vi "EF_DAQThread.vi"(9 "EF_DAQThread_Data":T1, 10 "EF_AllQRefs":T3, 11 "Exit":refnum<user-event>) -> ()   [LabVIEW 2017]
uses:
  Types/EF_AllQRefs.ctl
  Types/EF_GUIThread_QRef.ctl
  Types/EF_GUIThread_QData.ctl
  Types/EF_GUIThread_QCmds.ctl
  Types/EF_DAQThread_QRef.ctl
  Types/EF_DAQThread_QData.ctl
  Types/EF_DAQThread_QCmds.ctl
  Types/EF_DataProcThread_QRef.ctl
  Types/EF_DataProcThread_QData.ctl
  Types/EF_DataProcThread_QCmds.ctl
  Types/EF_AnalysisThread_QRef.ctl
  Types/EF_AnalysisThread_QData.ctl
  Types/EF_AnalysisThread_QCmds.ctl
  Types/EF_DAQThread_Data.ctl
  _lib/PQ/PicoHarp/PH_InitInfo.ctl
  _lib/PQ/PicoHarp/PH_MeasMode.ctl
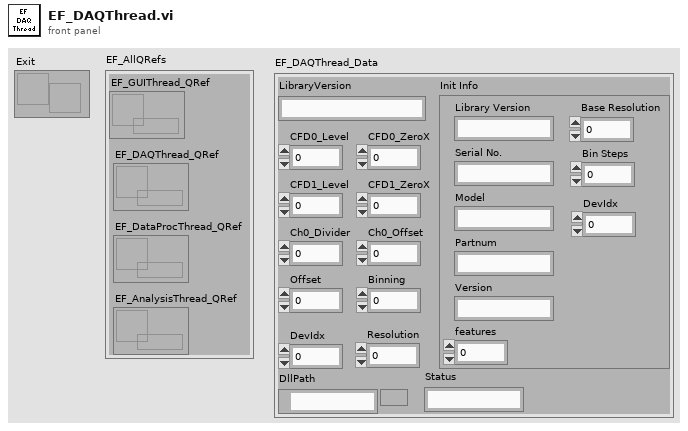
[diagram p1: front panel]
types:
  T1 = typedef "EF_DAQThread_Data.ctl" = cluster{"LibraryVersion":string, "CFD0_Level":i32, "CFD0_ZeroX":i32, "CFD1_Level":i32, "CFD1_ZeroX":i32, "Ch0_Divider":i32, "Ch0_Offset":i32, "Init Info":T2, "DevIdx":i32, "Offset":i32, "Binning":i32, "Resolution":dbl, "DllPath":path, "Status":string}
  T2 = typedef "PH_InitInfo.ctl" = cluster{"Library Version":string, "Serial No.":string, "Model":string, "Partnum":string, "Version":string, "features":i32, "Base Resolution":dbl, "Bin Steps":i32, "DevIdx":i32}
  T3 = typedef "EF_AllQRefs.ctl" = cluster{"EF_GUIThread_QRef":T4, "EF_DAQThread_QRef":T5, "EF_DataProcThread_QRef":T6, "EF_AnalysisThread_QRef":T7}
  T4 = typedef "EF_GUIThread_QRef.ctl" = refnum<queue>
  T5 = typedef "EF_DAQThread_QRef.ctl" = refnum<queue>
  T6 = typedef "EF_DataProcThread_QRef.ctl" = refnum<queue>
  T7 = typedef "EF_AnalysisThread_QRef.ctl" = refnum<queue>
  T8 = typedef "EF_DAQThread_QData.ctl" = cluster{"EF_DAQThread_Cmds":T9, "Parameter":i32[], "error in (no error)":errorcluster}
  T9 = typedef "EF_DAQThread_QCmds.ctl" = enum16{"Idle", "Init", "InitHW", "SetCFD0", "SetCFD1", "SetCh0Divider", "SetCh0Offset", "SetOffset", "SetBinning", "GetResolution", "GetRates", "StartMeas", "ReadFiFo", "StopMeas", "WriteStatus", "_Error_", "Exit"}
  T10 = typedef "EF_AnalysisThread_QData.ctl" = cluster{"Cmd":T11, "Histo":u32[], "DecayT0":dbl, "HistoRes":dbl, "TotalBinHistStart":u64, "TimeTraceRes":dbl, "Total bin":u64, "TickCount":u32, "LTThreshold":dbl, "TTLActivate":bool, "TTLDelay":dbl, "TTLWidth":dbl, "MinIntCounts":u32}
  T11 = typedef "EF_AnalysisThread_QCmds.ctl" = enum16{"Exit", "CalcAvgLT", "CalcDelay", "SetDecayT0", "SetHistoRes", "SetTimeTraceRes", "SetLTThreshold", "SetTTLActiv", "SetTTLDelay", "SetTTLWidth", "SetMinIntCounts"}
  T12 = typedef "EF_GUIThread_QData.ctl" = cluster{"Histo":u32[], "Rates":i32[], "Cmd":T13, "Res":dbl, "TimeTrace":u32[], "Bin":i32, "Status":string, "Total bin":u64, "AvgLTs":dbl[], "TotalBinsHistStart":u64[], "HistStartTimes":dbl[], "MinDelays":dbl[], "ShortDelay":bool, "Pending TTLs":i32, "error in (no error)":errorcluster, "DeltaT":dbl, "NumLTs":i32}
  T13 = typedef "EF_GUIThread_QCmds.ctl" = enum16{"_none_", "Res", "Histo", "TTrace", "Lifetime", "Rates", "Status", "ShortDelay", "_Error_"}
  T14 = typedef "EF_DataProcThread_QData.ctl" = cluster{"EF_DataProc_Cmds":T15, "nActual":i32, "Buffer":u32[], "TickCount":u32, "Param":i32}
  T15 = typedef "EF_DataProcThread_QCmds.ctl" = enum16{"Exit", "Proc", "Init", "SetShift", "SetThres"}
  T16 = typedef "PH_MeasMode.ctl" = i32
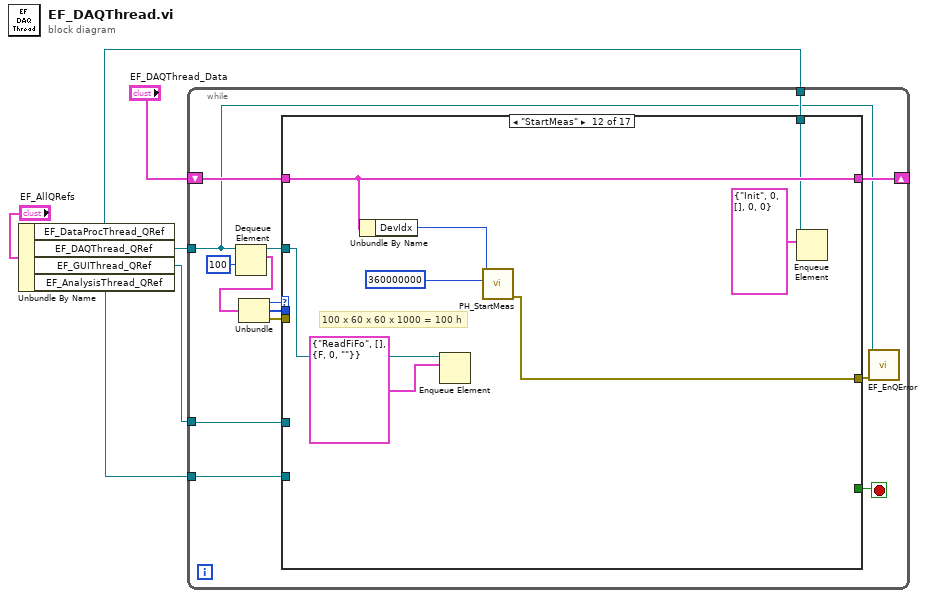
[diagram p0: block diagram]
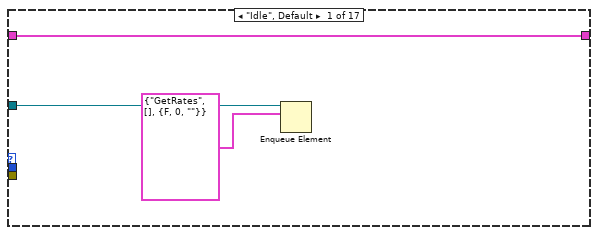
[diagram p2: hidden frame]
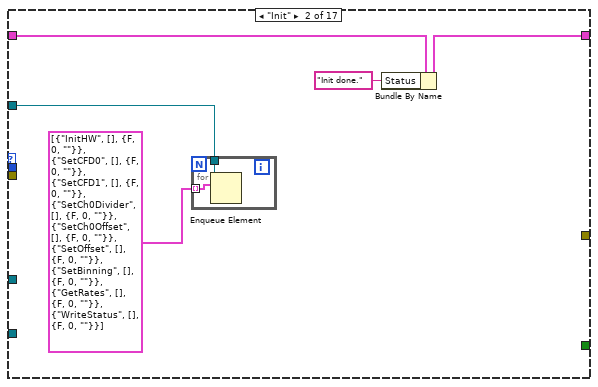
[diagram p3: hidden frame]
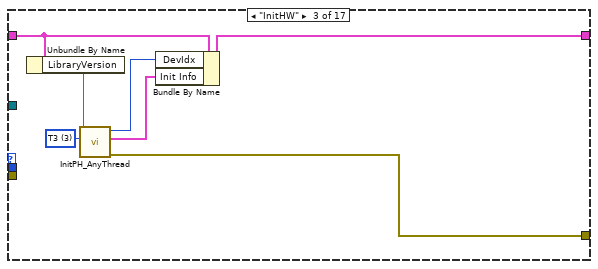
[diagram p4: hidden frame]
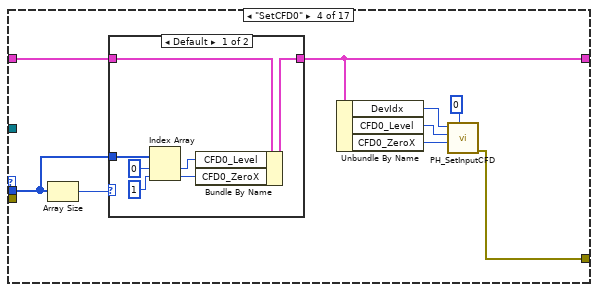
[diagram p5: hidden frame]
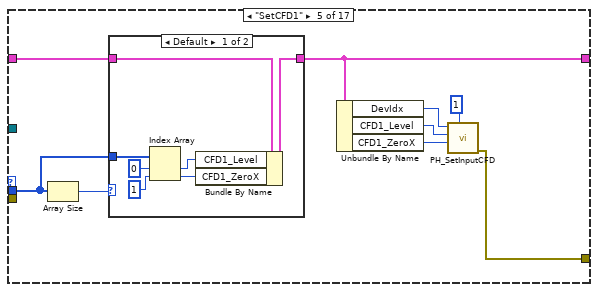
[diagram p7: hidden frame]
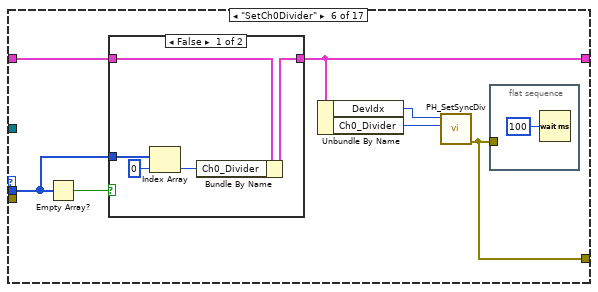
[diagram p9: hidden frame]
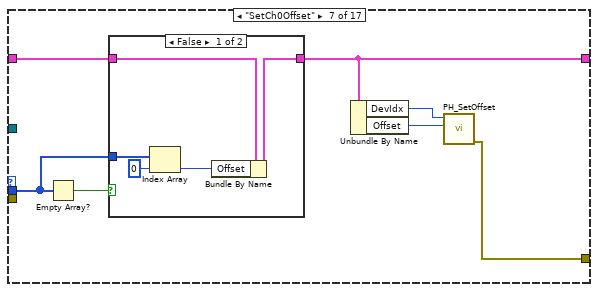
[diagram p11: hidden frame]
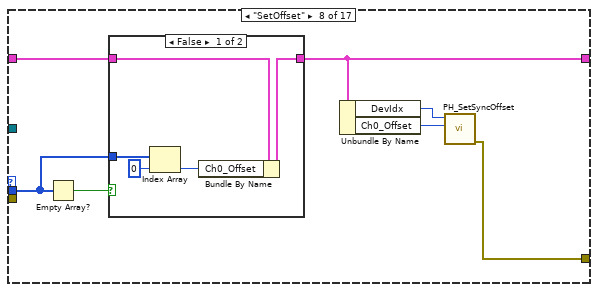
[diagram p13: hidden frame]
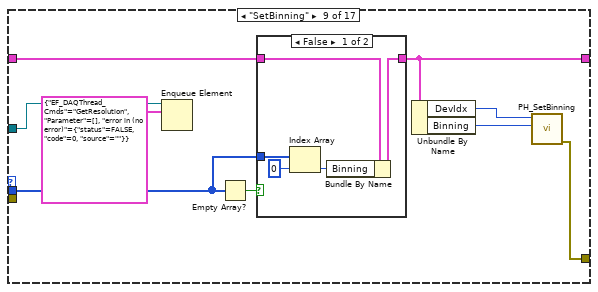
[diagram p15: hidden frame]
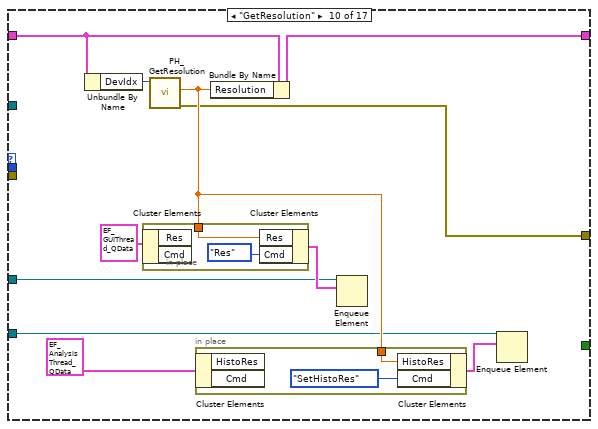
[diagram p17: hidden frame]
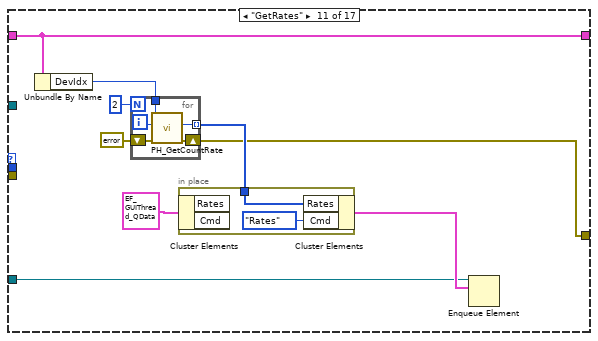
[diagram p18: hidden frame]
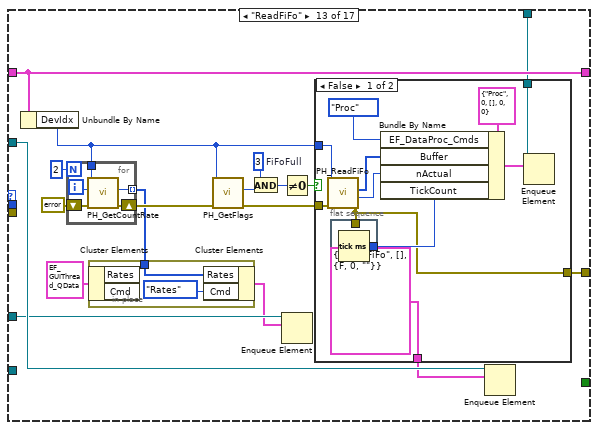
[diagram p19: hidden frame]
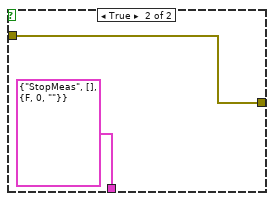
[diagram p20: hidden frame]
diagram:
  n1 = Unbundle By Name("EF_AllQRefs") -> ("EF_DataProcThread_QRef"=w3:T6, "EF_DAQThread_QRef"=w1:T5, "EF_GUIThread_QRef"=w4:T4, "EF_AnalysisThread_QRef"=w2:T7)
  n2 = while {
    tunnel: w1 -> [w8]
    shift-right: [w15] -> _
    shift-left: "EF_DAQThread_Data" -> [w14]
    tunnel: w4 -> [w12]
    tunnel: w3 -> [w11]
    tunnel: w2 -> [w10]
    stop <- w18 stop-if-true
    n3 = Dequeue Element(queue=w8, timeout in ms (-1)=100) -> (queue out=w16:T5, element=w20:T8)  [unwired: 1 in, 2 out]
    n4 = Unbundle(w20) -> ("EF_DAQThread_Cmds"=w19:T9, "Parameter"=w13:i32[], "error in (no error)"=w7:errorcluster)
    n5 = case shown="\"StartMeas\"" w19 {
      tunnel: [_ _ _ _ _ _ _ _ _ _ _ _ _ _ _ _ TRUE] -> w18
      tunnel: w16 -> [w22 w28 _ _ _ _ _ _ w114 _ _ w161 w177 w207 _ w232 w245]
      tunnel: [w23 w26 w33 w42 w59 w75 w89 w102 w117 w135 w150 w165 w183 w210 w218 w233 w244] -> w15
      tunnel: w14 -> [w23 w24 w34 w46 w63 w78 w92 w105 w120 w136 w150 w165 w183 w210 w218 w233 w244]
      tunnel: w13 -> [_ _ _ w45 w62 w77 w91 w104 w119 _ _ _ _ _ _ _ _]
      tunnel: w12 -> [_ _ _ _ _ _ _ _ _ w132 w147 _ w173 _ w219 w231 w241]
      tunnel: w11 -> [_ _ _ _ _ _ _ _ _ _ _ w162 w172 _ _ _ w242]
      tunnel: w10 -> [_ _ _ _ _ _ _ _ _ w128 _ _ _ _ _ _ _]
      tunnel: [_ _ w31 w38 w55 w72 w86 w99 w112 w127 w142 w159 w166 w205 _ _ w234] -> w9
      tunnel: w7 -> [_ _ _ _ _ _ _ _ _ _ _ _ _ _ _ w229 _]
      frame "Idle", Default {
        n6 = Enqueue Element(queue=w22, element=T8 {"EF_DAQThread_Cmds"=enum."GetRates", "Parameter"=[], "error in (no error)"={"status"=FALSE, "code"=0, "source"=""}}) -> ()  [unwired: 2 in, 3 out]
      }
      frame "Init" {
        n7 = for {
          tunnel: w28 -> [w30]
          tunnel: T8[] [{"EF_DAQThread_Cmds"=enum."InitHW", "Parameter"=[], "error in (no error)"={"status"=FALSE, "code"=0, "source"=""}}, {"EF_DAQThread_Cmds"=enum."SetCFD0", "Parameter"=[], "error in (no error)"={"status"=FALSE, "code"=0, "source"=""}}, {"EF_DAQThread_Cmds"=enum."SetCFD1", "Parameter"=[], "error in (no error)"={"status"=FALSE, "code"=0, "source"=""}}, {"EF_DAQThread_Cmds"=enum."SetCh0Divider", "Parameter"=[], "error in (no error)"={"status"=FALSE, "code"=0, "source"=""}}, {"EF_DAQThread_Cmds"=enum."SetCh0Offset", "Parameter"=[], "error in (no error)"={"status"=FALSE, "code"=0, "source"=""}}, {"EF_DAQThread_Cmds"=enum."SetOffset", "Parameter"=[], "error in (no error)"={"status"=FALSE, "code"=0, "source"=""}}, {"EF_DAQThread_Cmds"=enum."SetBinning", "Parameter"=[], "error in (no error)"={"status"=FALSE, "code"=0, "source"=""}}, {"EF_DAQThread_Cmds"=enum."GetRates", "Parameter"=[], "error in (no error)"={"status"=FALSE, "code"=0, "source"=""}}, {"EF_DAQThread_Cmds"=enum."WriteStatus", "Parameter"=[], "error in (no error)"={"status"=FALSE, "code"=0, "source"=""}}] -> [w29] mode=indexing
          n8 = Enqueue Element(queue=w30, element=w29) -> ()  [unwired: 2 in, 3 out]
        }
        n9 = Bundle By Name(cluster=w24, "Status"="Init done.") -> (w26:T1)
      }
      frame "InitHW" {
        w36 = T16 3 items=["Histo"=0, "T2"=2, "T3"=3] ("mode")
        n10 = Unbundle By Name(w34) -> ("LibraryVersion"=w37:string)
        n11 = call "InitPH_AnyThread.vi"("mode"=w36, "Library Version"=w37) -> ("Error"=w31:errorcluster, "Init Info"=w35:T2, "DevIdx"=w32:i32)  [unwired: 7 in]
        n12 = Bundle By Name(cluster=w34, "DevIdx"=w32, "Init Info"=w35) -> (w33:T1)
      }
      frame "SetCFD0" {
        n13 = Array Size(array=w45) -> (size(s)=w44:i32)
        n14 = case shown="Default" w44 {
          tunnel: w46 -> [w53 w54]
          tunnel: [w52 w54] -> w42
          tunnel: w45 -> [w51 _]
          frame Default {
            n15 = Index Array(array=w51, index #1=0 ("index"), index #2=1 ("index")) -> (element #1=w50:i32, element #2=w49:i32)
            n16 = Bundle By Name(cluster=w53, "CFD0_Level"=w50, "CFD0_ZeroX"=w49) -> (w52:T1)
          }
          frame 0, 1 {
          }
        }
        n17 = Unbundle By Name(w42) -> ("DevIdx"=w41:i32, "CFD0_Level"=w40:i32, "CFD0_ZeroX"=w39:i32)
        n18 = call "PH_SetInputCFD.vi"("CFD Channel"=0, "CFD ZeroCross"=w39, "CFD Level"=w40, "devidx"=w41) -> ("error out"=w38:errorcluster)  [unwired: 6 in, 1 out]
      }
      frame "SetCFD1" {
        n19 = Array Size(array=w62) -> (size(s)=w61:i32)
        n20 = case shown="Default" w61 {
          tunnel: w63 -> [w70 w71]
          tunnel: [w69 w71] -> w59
          tunnel: w62 -> [w68 _]
          frame Default {
            n21 = Index Array(array=w68, index #1=0 ("index"), index #2=1 ("index")) -> (element #1=w67:i32, element #2=w66:i32)
            n22 = Bundle By Name(cluster=w70, "CFD1_Level"=w67, "CFD1_ZeroX"=w66) -> (w69:T1)
          }
          frame 0, 1 {
          }
        }
        n23 = Unbundle By Name(w59) -> ("DevIdx"=w58:i32, "CFD1_Level"=w57:i32, "CFD1_ZeroX"=w56:i32)
        n24 = call "PH_SetInputCFD.vi"("CFD Channel"=1, "CFD ZeroCross"=w56, "CFD Level"=w57, "devidx"=w58) -> ("error out"=w55:errorcluster)  [unwired: 6 in, 1 out]
      }
      frame "SetCh0Divider" {
        n25 = Empty Array?(array=w77) -> (empty?=w76:bool)
        n26 = case shown="False" w76 {
          tunnel: w78 -> [w84 w85]
          tunnel: [w83 w85] -> w75
          tunnel: w77 -> [w82 _]
          frame False {
            n27 = Index Array(array=w82, index=0) -> (element=w81:i32)
            n28 = Bundle By Name(cluster=w84, "Ch0_Divider"=w81) -> (w83:T1)
          }
          frame True {
          }
        }
        n29 = Unbundle By Name(w75) -> ("DevIdx"=w73:i32, "Ch0_Divider"=w74:i32)
        n30 = call "PH_SetSyncDiv.vi"("SyncDivider"=w74, "devidx"=w73) -> ("error out"=w72:errorcluster)  [unwired: 8 in, 1 out]
        n31 = flat-sequence {
          tunnel: w72 -> [_]
          frame #0 {
            n32 = Wait (ms)(milliseconds to wait=u32 100) -> ()  [unwired: 1 out]
          }
        }
      }
      frame "SetCh0Offset" {
        n33 = Empty Array?(array=w91) -> (empty?=w90:bool)
        n34 = case shown="False" w90 {
          tunnel: w92 -> [w97 w98]
          tunnel: [w96 w98] -> w89
          tunnel: w91 -> [w95 _]
          frame False {
            n35 = Index Array(array=w95, index=0) -> (element=w94:i32)
            n36 = Bundle By Name(cluster=w97, "Offset"=w94) -> (w96:T1)
          }
          frame True {
          }
        }
        n37 = Unbundle By Name(w89) -> ("DevIdx"=w87:i32, "Offset"=w88:i32)
        n38 = call "PH_SetOffset.vi"("Offset"=w88, "devidx"=w87) -> ("error out"=w86:errorcluster)  [unwired: 8 in, 1 out]
      }
      frame "SetOffset" {
        n39 = Empty Array?(array=w104) -> (empty?=w103:bool)
        n40 = case shown="False" w103 {
          tunnel: w105 -> [w110 w111]
          tunnel: [w109 w111] -> w102
          tunnel: w104 -> [w108 _]
          frame False {
            n41 = Index Array(array=w108, index=0) -> (element=w107:i32)
            n42 = Bundle By Name(cluster=w110, "Ch0_Offset"=w107) -> (w109:T1)
          }
          frame True {
          }
        }
        n43 = Unbundle By Name(w102) -> ("DevIdx"=w100:i32, "Ch0_Offset"=w101:i32)
        n44 = call "PH_SetSyncOffset.vi"("Offset"=w101, "devidx"=w100) -> ("error out"=w99:errorcluster)  [unwired: 8 in, 1 out]
      }
      frame "SetBinning" {
        n45 = Enqueue Element(queue=w114, element=T8 {"EF_DAQThread_Cmds"=enum."GetResolution", "Parameter"=[], "error in (no error)"={"status"=FALSE, "code"=0, "source"=""}}) -> ()  [unwired: 2 in, 3 out]
        n46 = Empty Array?(array=w119) -> (empty?=w118:bool)
        n47 = case shown="False" w118 {
          tunnel: w120 -> [w125 w126]
          tunnel: [w124 w126] -> w117
          tunnel: w119 -> [w123 _]
          frame False {
            n48 = Index Array(array=w123, index=0) -> (element=w122:i32)
            n49 = Bundle By Name(cluster=w125, "Binning"=w122) -> (w124:T1)
          }
          frame True {
          }
        }
        n50 = Unbundle By Name(w117) -> ("DevIdx"=w115:i32, "Binning"=w116:i32)
        n51 = call "PH_SetBinning.vi"("Binning"=w116, "devidx"=w115) -> ("error out"=w112:errorcluster)  [unwired: 8 in, 1 out]
      }
      frame "GetResolution" {
        n52 = Unbundle By Name(w136) -> ("DevIdx"=w137:i32)
        n53 = call "PH_GetResolution.vi"("devidx"=w137) -> ("error out"=w127:errorcluster, "resolution"=w130:dbl)  [unwired: 8 in, 1 out]
        n54 = in-place {
          in-place-border: w130 -> [w141]
          n55 = in-place-cluster #1(T12 {"Histo"=[], "Rates"=[], "Cmd"=enum."_none_", "Res"=0.0, "TimeTrace"=[], "Bin"=0, "Status"="", "Total bin"=0, "AvgLTs"=[], "TotalBinsHistStart"=[], "HistStartTimes"=[], "MinDelays"=[], "ShortDelay"=FALSE, "Pending TTLs"=0, "error in (no error)"={"status"=FALSE, "code"=0, "source"=""}, "DeltaT"=0.0, "NumLTs"=0} ("EF_VisualData")) -> ()  [unwired: 2 out]
          n56 = in-place-cluster #1("Res"=w141, "Cmd"=EF_GUIThread_QCmds."Res") -> (w133:T12)
        }
        n57 = in-place {
          in-place-border: w130 -> [w139]
          n58 = in-place-cluster #2(T10 {"Cmd"=enum."Exit", "Histo"=[], "DecayT0"=0.0, "HistoRes"=0.0, "TotalBinHistStart"=0, "TimeTraceRes"=0.0, "Total bin"=0, "TickCount"=0, "LTThreshold"=0.0, "TTLActivate"=FALSE, "TTLDelay"=0.0, "TTLWidth"=0.0, "MinIntCounts"=0} ("element")) -> ()  [unwired: 2 out]
          n59 = in-place-cluster #2("HistoRes"=w139, "Cmd"=EF_AnalysisThread_QCmds."SetHistoRes") -> (w129:T10)
        }
        n60 = Bundle By Name(cluster=w136, "Resolution"=w130) -> (w135:T1)
        n61 = Enqueue Element(queue=w132, element=w133) -> ()  [unwired: 2 in, 3 out]
        n62 = Enqueue Element(queue=w128, element=w129) -> ()  [unwired: 2 in, 3 out]
      }
      frame "GetRates" {
        n63 = Unbundle By Name(w150) -> ("DevIdx"=w145:i32)
        n64 = for {
          N: 2 -> [_]
          tunnel: w145 -> [w153]
          shift-right: [w154] -> w142
          shift-left: errorcluster {"status"=FALSE, "code"=0, "source"=""} ("error out") -> [w155]
          tunnel: [w151] -> w144 mode=indexing
          i -> [w152]
          n65 = call "PH_GetCountRate.vi"("error in (no error)"=w155, "Channel"=w152, "devidx"=w153) -> ("error out"=w154:errorcluster, "rate"=w151:i32)  [unwired: 6 in, 1 out]
        }
        n66 = in-place {
          in-place-border: w144 -> [w157]
          n67 = in-place-cluster #3(T12 {"Histo"=[], "Rates"=[], "Cmd"=enum."_none_", "Res"=0.0, "TimeTrace"=[], "Bin"=0, "Status"="", "Total bin"=0, "AvgLTs"=[], "TotalBinsHistStart"=[], "HistStartTimes"=[], "MinDelays"=[], "ShortDelay"=FALSE, "Pending TTLs"=0, "error in (no error)"={"status"=FALSE, "code"=0, "source"=""}, "DeltaT"=0.0, "NumLTs"=0} ("EF_VisualData")) -> ()  [unwired: 2 out]
          n68 = in-place-cluster #3("Rates"=w157, "Cmd"=EF_GUIThread_QCmds."Rates") -> (w148:T12)
        }
        n69 = Enqueue Element(queue=w147, element=w148) -> ()  [unwired: 2 in, 3 out]
      }
      frame "StartMeas" {
        # "100 x 60 x 60 x 1000 = 100 h"
        n70 = Unbundle By Name(w165) -> ("DevIdx"=w164:i32)
        n71 = Enqueue Element(queue=w161, element=T8 {"EF_DAQThread_Cmds"=enum."ReadFiFo", "Parameter"=[], "error in (no error)"={"status"=FALSE, "code"=0, "source"=""}}) -> ()  [unwired: 2 in, 3 out]
        n72 = call "PH_StartMeas.vi"("Acquisition time"=360000000 ("Acqu. Time"), "devidx"=w164) -> ("error out"=w159:errorcluster)  [unwired: 8 in, 1 out]
        n73 = Enqueue Element(queue=w162, element=T14 {"EF_DataProc_Cmds"=enum."Init", "nActual"=0, "Buffer"=[], "TickCount"=0, "Param"=0}) -> ()  [unwired: 2 in, 3 out]
      }
      frame "ReadFiFo" {
        w180 = 3  # FiFoFull
        n74 = Unbundle By Name(w183) -> ("DevIdx"=w174:i32)
        n75 = for {
          N: 2 -> [_]
          tunnel: w174 -> [w188]
          shift-right: [w189] -> w175
          shift-left: errorcluster {"status"=FALSE, "code"=0, "source"=""} ("error out") -> [w190]
          tunnel: [w186] -> w169 mode=indexing
          i -> [w187]
          n76 = call "PH_GetCountRate.vi"("error in (no error)"=w190, "Channel"=w187, "devidx"=w188) -> ("error out"=w189:errorcluster, "rate"=w186:i32)  [unwired: 6 in, 1 out]
        }
        n77 = in-place {
          in-place-border: w169 -> [w185]
          n78 = in-place-cluster #4(T12 {"Histo"=[], "Rates"=[], "Cmd"=enum."_none_", "Res"=0.0, "TimeTrace"=[], "Bin"=0, "Status"="", "Total bin"=0, "AvgLTs"=[], "TotalBinsHistStart"=[], "HistStartTimes"=[], "MinDelays"=[], "ShortDelay"=FALSE, "Pending TTLs"=0, "error in (no error)"={"status"=FALSE, "code"=0, "source"=""}, "DeltaT"=0.0, "NumLTs"=0} ("EF_VisualData")) -> ()  [unwired: 2 out]
          n79 = in-place-cluster #4("Rates"=w185, "Cmd"=EF_GUIThread_QCmds."Rates") -> (w168:T12)
        }
        n80 = call "PH_GetFlags.vi"("error in (no error)"=w175, "devidx"=w174) -> ("error out"=w178:errorcluster, "flags"=w181:i32)  [unwired: 7 in, 1 out]
        n81 = And(x=w180, y=w181) -> (x .and. y?=w182:i32)
        n82 = Not Equal To 0?(x=w182) -> (x != 0?=w179:bool)
        n83 = Enqueue Element(queue=w173, element=w168) -> ()  [unwired: 2 in, 3 out]
        n84 = case shown="False" w179 {
          tunnel: w174 -> [w201 _]
          tunnel: w178 -> [w200 w203]
          tunnel: [T8 {"EF_DAQThread_Cmds"=enum."ReadFiFo", "Parameter"=[], "error in (no error)"={"status"=FALSE, "code"=0, "source"=""}} ("element") T8 {"EF_DAQThread_Cmds"=enum."StopMeas", "Parameter"=[], "error in (no error)"={"status"=FALSE, "code"=0, "source"=""}} ("element")] -> w176
          tunnel: w172 -> [w192 _]
          tunnel: [w191 w203] -> w166
          frame False {
            n85 = call "PH_ReadFiFo.vi"("error in (no error)"=w200, "devidx"=w201) -> ("error out"=w191:errorcluster, "nactual"=w196:i32, "buffer"=w197:u32[])  [unwired: 6 in, 1 out]
            n86 = flat-sequence {
              tunnel: w191 -> [_]
              tunnel: [w202] -> w195
              frame #0 {
                n87 = Tick Count (ms)() -> (millisecond timer value=w202:u32)
              }
            }
            n88 = Bundle By Name(cluster=T14 {"EF_DataProc_Cmds"=enum."Proc", "nActual"=0, "Buffer"=[], "TickCount"=0, "Param"=0} ("element"), "EF_DataProc_Cmds"=EF_DataProcThread_QCmds."Proc", "Buffer"=w197, "nActual"=w196, "TickCount"=w195) -> (w193:T14)
            n89 = Enqueue Element(queue=w192, element=w193) -> ()  [unwired: 2 in, 3 out]
          }
          frame True {
          }
        }
        n90 = Enqueue Element(queue=w177, element=w176) -> ()  [unwired: 2 in, 3 out]
      }
      frame "StopMeas" {
        n91 = Flush Queue(queue=w207) -> (remaining elements=w208:T8[])  [unwired: 1 in, 2 out]
        n92 = Unbundle By Name(w210) -> ("DevIdx"=w209:i32)
        n93 = for {
          tunnel: w208 -> [w216] mode=indexing
          tunnel: [w213] -> w206
          stop <- w213 stop-if-true
          n94 = Unbundle By Name(w216) -> ("EF_DAQThread_Cmds"=w215:T9)
          n95 = Equal?(x=w215, y=EF_DAQThread_QCmds."Exit" ("EF_DAQThread_Cmds")) -> (x = y?=w213:bool)
        }
        n96 = call "PH_StopMeas.vi"("devidx"=w209) -> ("error out"=w205:errorcluster)  [unwired: 9 in, 1 out]
        n97 = case shown="False" w206 {
          tunnel: w207 -> [_ w212]
          frame False {
          }
          frame True {
            n98 = Enqueue Element(queue=w212, element=T8 {"EF_DAQThread_Cmds"=enum."Exit", "Parameter"=[], "error in (no error)"={"status"=FALSE, "code"=0, "source"=""}}) -> ()  [unwired: 2 in, 3 out]
          }
        }
      }
      frame "WriteStatus" {
        n99 = Unbundle By Name(w218) -> ("Status"=w217:string)
        n100 = in-place {
          in-place-border: w217 -> [w222]
          n101 = in-place-cluster #5(T12 {"Histo"=[], "Rates"=[], "Cmd"=enum."_none_", "Res"=0.0, "TimeTrace"=[], "Bin"=0, "Status"="", "Total bin"=0, "AvgLTs"=[], "TotalBinsHistStart"=[], "HistStartTimes"=[], "MinDelays"=[], "ShortDelay"=FALSE, "Pending TTLs"=0, "error in (no error)"={"status"=FALSE, "code"=0, "source"=""}, "DeltaT"=0.0, "NumLTs"=0} ("EF_VisualData")) -> ()  [unwired: 2 out]
          n102 = in-place-cluster #5("Status"=w222, "Cmd"=EF_GUIThread_QCmds."Status") -> (w221:T12)
        }
        n103 = Enqueue Element(queue=w219, element=w221) -> ()  [unwired: 2 in, 3 out]
      }
      frame "_Error_" {
        n104 = Flush Queue(queue=w232) -> (queue out=w224:T5, error out=w226:errorcluster)  [unwired: 1 in, 1 out]
        n105 = Preview Queue Element(queue=w224, error in (no error)=w226) -> ()  [unwired: 1 in, 4 out]
        n106 = Unbundle By Name(w233) -> ("DevIdx"=w225:i32)
        n107 = Bundle By Name(cluster=T12 {"Histo"=[], "Rates"=[], "Cmd"=enum."_none_", "Res"=0.0, "TimeTrace"=[], "Bin"=0, "Status"="", "Total bin"=0, "AvgLTs"=[], "TotalBinsHistStart"=[], "HistStartTimes"=[], "MinDelays"=[], "ShortDelay"=FALSE, "Pending TTLs"=0, "error in (no error)"={"status"=FALSE, "code"=0, "source"=""}, "DeltaT"=0.0, "NumLTs"=0} ("EF_VisualData"), "Cmd"=EF_GUIThread_QCmds."_Error_", "error in (no error)"=w229) -> (w228:T12)
        n108 = call "PH_StopMeas.vi"("devidx"=w225) -> ()  [unwired: 9 in, 2 out]
        n109 = Enqueue Element(queue=w231, element=w228) -> ()  [unwired: 2 in, 3 out]
      }
      frame "Exit" {
        n110 = Unbundle By Name(w244) -> ("DevIdx"=w243:i32)
        n111 = Release Queue(queue=w245) -> ()  [unwired: 2 in, 3 out]
        n112 = while {
          tunnel: w241 -> [w251]
          tunnel: [w250] -> w240
          tunnel: [errorcluster {"status"=FALSE, "code"=0, "source"=""} ("error in (no error)")] -> w237
          i -> [w256]
          stop <- w252 stop-if-true
          n113 = Get Queue Status(queue=w251) -> (queue out=w250:T4, # elements in queue=w258:i32)  [unwired: 2 in, 6 out]
          n114 = Wait (ms)(milliseconds to wait=u32 100) -> ()  [unwired: 1 out]
          n115 = Greater Or Equal?(x=w256, y=20) -> (x >= y?=w254:bool)
          n116 = Equal To 0?(x=w258) -> (x = 0?=w253:bool)
          n117 = Or(x=w254, y=w253) -> (x .or. y?=w252:bool)
        }
        n118 = call "PH_CloseDevice.vi"("devidx"=w243) -> ("error out"=w234:errorcluster)  [unwired: 9 in, 1 out]
        n119 = Generate User Event(user event="Exit", event data cluster=TRUE ("event data"), error in=w237) -> (error out=w236:errorcluster)  [unwired: 1 in, 1 out]
        n120 = flat-sequence {
          tunnel: w236 -> [w247]
          tunnel: [w247] -> w235
          frame #0 {
            n121 = Wait (ms)(milliseconds to wait=u32 100) -> ()  [unwired: 1 out]
          }
        }
        n122 = Release Queue(queue=w240, error in (no error)=w235) -> ()  [unwired: 1 in, 3 out]
        n123 = Release Queue(queue=w242) -> ()  [unwired: 2 in, 3 out]
      }
    }
    n124 = call "EF_EnQError.vi"("error in (no error)"=w9, "Queue in"=w8) -> ()  [unwired: 10 in]
  }
